vi "tcp data queue array back to comma separated.vi"(10 "TCP subscriptions info":T1, 11 "All data":string[][](array[string])) -> (3 "Comma separated":string[](array[string]))   [LabVIEW 2020]
uses:
  Shared/GUI_Template/TCP subscription info cluster.ctl
panel:
  out "all the variables":string[](array[string])
  out "Devices repeated for each variable":string[](array[string])
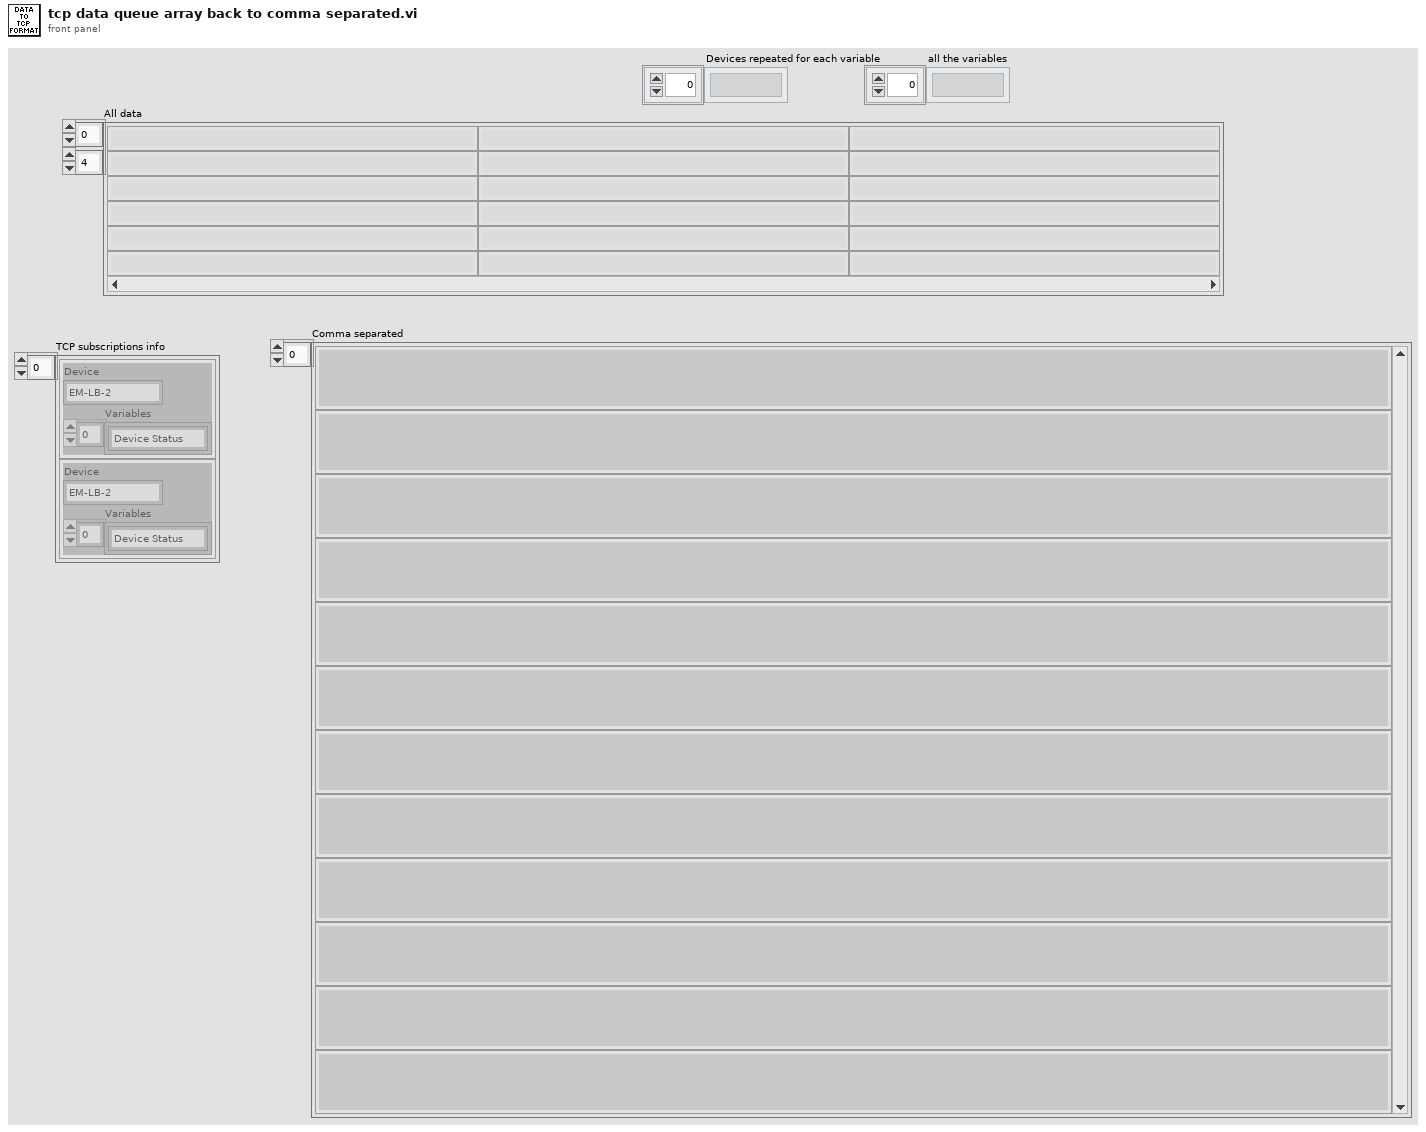
[diagram p1: front panel]
types:
  T1 = typedef "TCP subscription info cluster.ctl" = cluster{"Device":string, "Variables":string[]}[]
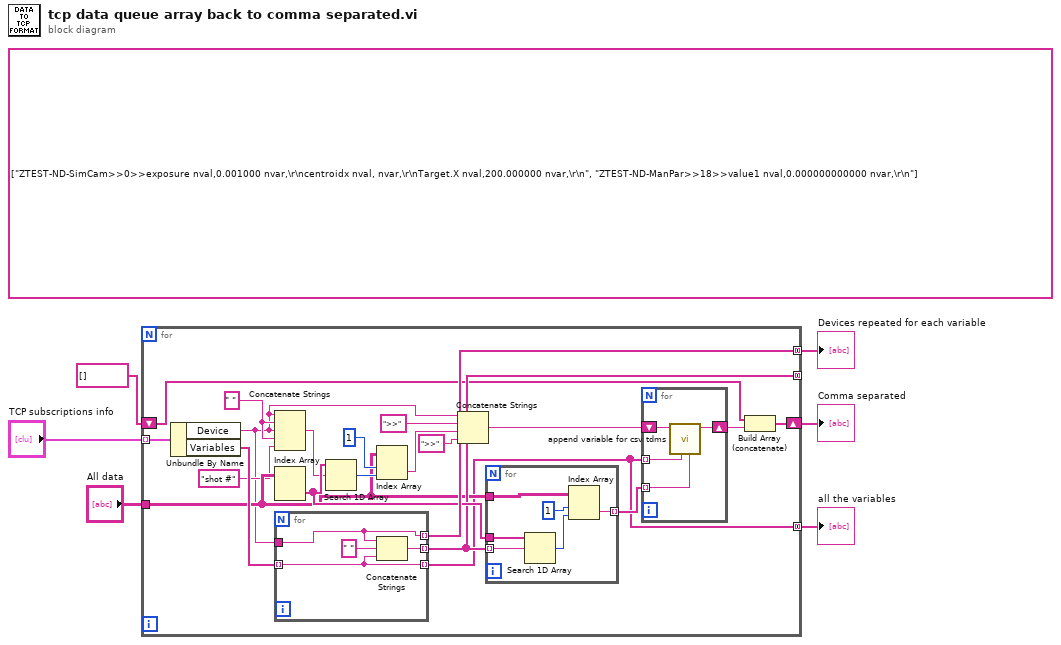
[diagram p0: block diagram]
diagram:
  (unwired) string[] ["ZTEST-ND-SimCam>>0>>exposure nval,0.001000 nvar,\r\ncentroidx nval, nvar,\r\nTarget.X nval,200.000000 nvar,\r\n", "ZTEST-ND-ManPar>>18>>value1 nval,0.000000000000 nvar,\r\n"] ("Scan data in")
  n1 = for {
    tunnel: "TCP subscriptions info" -> [w27] mode=indexing
    tunnel: [w21] -> _ mode=concatenating
    tunnel: [w25] -> w5 mode=concatenating
    tunnel: [w15] -> w4 mode=concatenating
    tunnel: "All data" -> [w20]
    shift-right: [w7] -> w1
    shift-left: string[] [] ("Scan data out") -> [w9]
    w17 = " " ("string")
    n2 = Unbundle By Name(w27) -> ("Device"=w12:string, "Variables"=w26:string[])
    n3 = Concatenate Strings(w12, w17, w12, w17, "shot #" ("string")) -> (w18:string)
    n4 = Index Array(array=w20) -> (element=w24:string[])  [unwired: 2 in]
    n5 = for {
      tunnel: w12 -> [w39]
      tunnel: w26 -> [w38] mode=indexing
      tunnel: [w40] -> w21 mode=indexing
      tunnel: [w39] -> w25 mode=indexing
      tunnel: [w38] -> w15 mode=indexing
      n6 = Concatenate Strings(w39, " " ("string"), w38) -> (w40:string)
    }
    n7 = Search 1D Array(1D array=w24, element=w18) -> (index of element=w22:i32)  [unwired: 1 in]
    n8 = Index Array(array=w20, index (row)=1, index (col)=w22) -> (element=w11:string)
    n9 = Concatenate Strings(w12, ">>" ("string"), w11, ">>" ("string")) -> (w10:string)
    n10 = for {
      tunnel: w24 -> [w37]
      tunnel: w21 -> [w36] mode=indexing
      tunnel: w20 -> [w35]
      tunnel: [w32] -> w19 mode=indexing
      n11 = Search 1D Array(1D array=w37, element=w36) -> (index of element=w33:i32)  [unwired: 1 in]
      n12 = Index Array(array=w35, index (row)=1, index (col)=w33) -> (element=w32:string)
    }
    n13 = for {
      tunnel: w15 -> [w29] mode=indexing
      tunnel: w19 -> [w28] mode=indexing
      shift-right: [w31] -> w8
      shift-left: w10 -> [w30]
      n14 = call "append variable for csv tdms.vi"("variable value"=w28, "variable name"=w29, "Input string"=w30) -> ("output string"=w31:string)  [unwired: 8 in]
    }
    n15 = Build Array (concatenate)(w9, w8) -> (w7:string[])
  }
  "Comma separated" <- w1
  "Devices repeated for each variable" <- w5
  "all the variables" <- w4
